vi "Datasheet Yield Result.vi"(6 "Connection Refnum":T1, 8 "error in (no error)":errorcluster, 10 "Yield Results":T3[](array[typedef]), 11 "Selected Test Type":string) -> (0 "error out":errorcluster, 3 "Key Array Out":T2)   [LabVIEW 2011]
uses:
  CGI Yield Results.ctl
  Addons/internet/utils/keyedarr.llb/Keyed Array.ctl
  SI.LIB/ODBC/SQL Controls/Connection Refnum.ctl
  Addons/internet/utils/strutil.llb/Case Matching.ctl
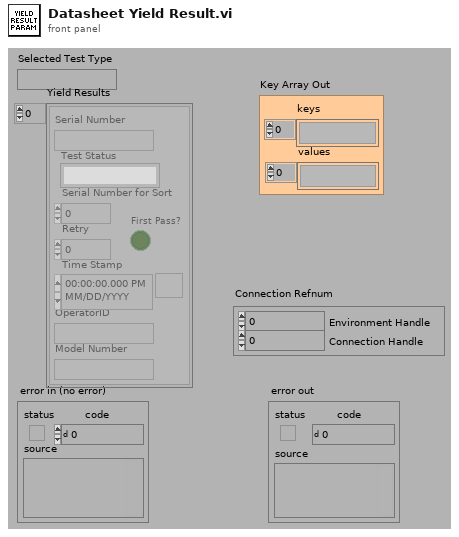
[diagram p1: front panel]
types:
  T1 = typedef "Connection Refnum.ctl" = cluster{"Environment Handle":i32, "Connection Handle":i32}
  T2 = typedef "Keyed Array.ctl" = cluster{"keys":string[], "values":string[]}
  T3 = typedef "CGI Yield Results.ctl" = cluster{"Model Number":string, "Serial Number for Sort":i32, "Serial Number":string, "Test Status":string, "Time Stamp":timestamp, "OperatorID":string, "Retry":i32, "First Pass?":bool}
  T4 = typedef "Case Matching.ctl" = enum16{"a != A", "a == A", "system"}
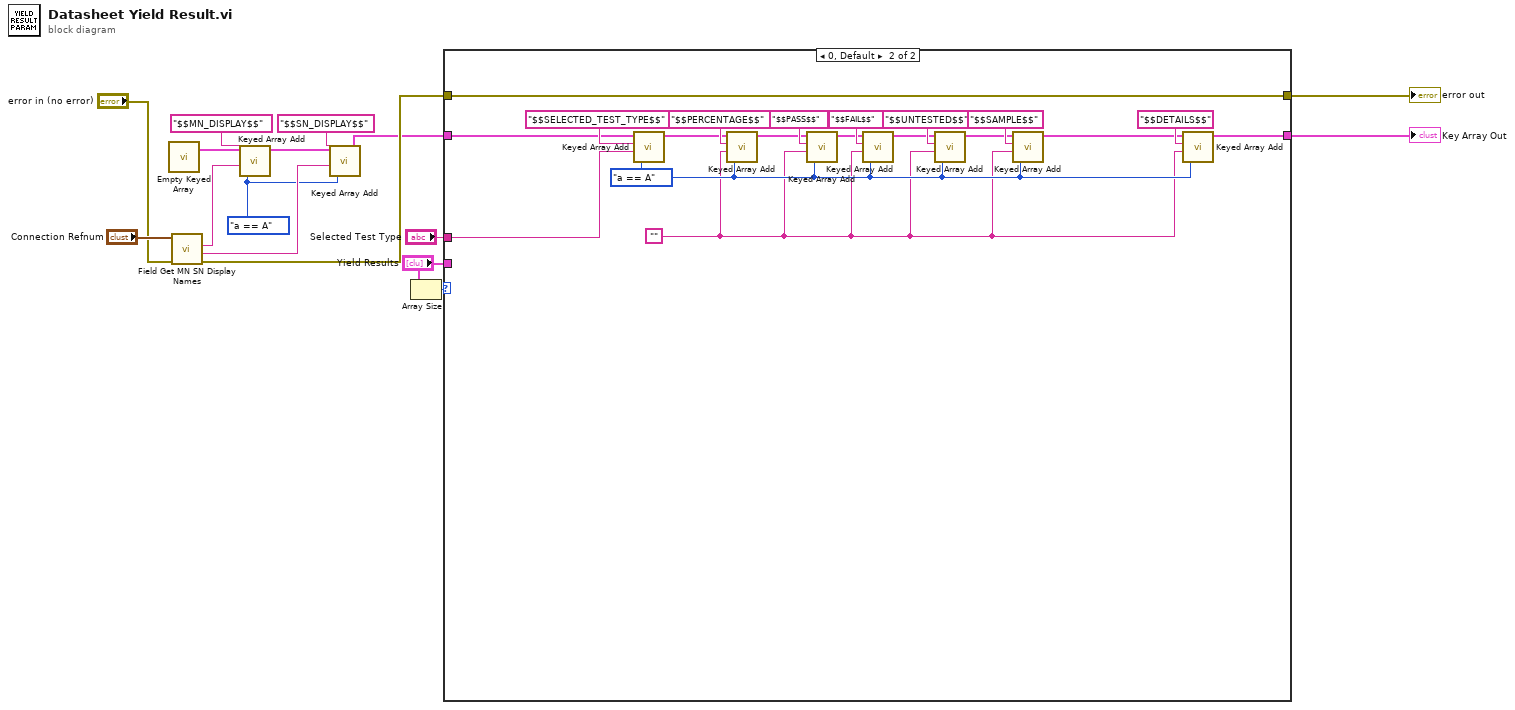
[diagram p0: block diagram]
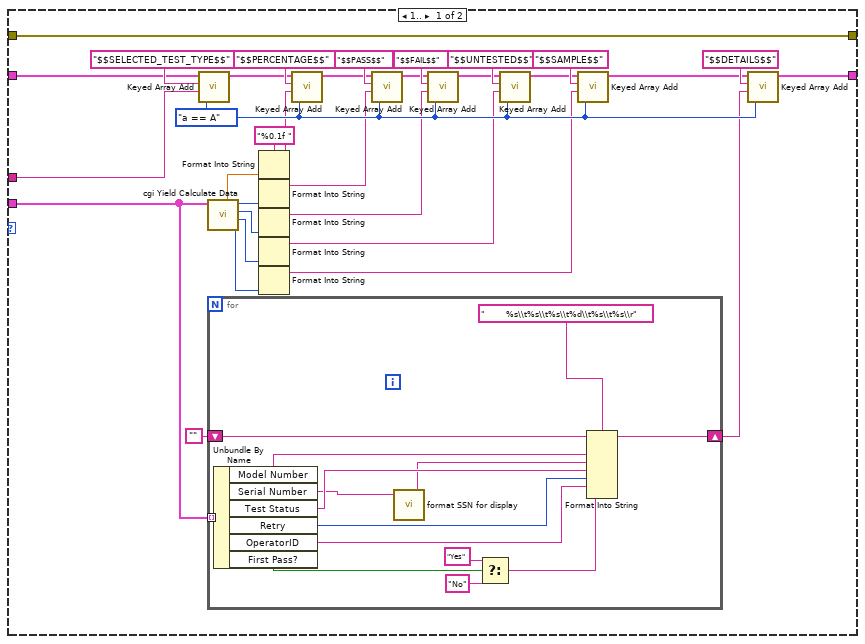
[diagram p2: hidden frame]
diagram:
  w6 = Case_Matching."a == A" ("case matching (sensitive)")
  n1 = call "Empty Keyed Array.vi"() -> ("empty keyed array"=w5:T2)  [unwired: 3 out]
  n2 = call "Field Get MN SN Display Names.vi"("error in (no error)"="error in (no error)", "Connection Refnum"="Connection Refnum") -> ("error out"=w2:errorcluster, "Serial Number Display Name"=w7:string, "Model Number Display Name"=w8:string)  [unwired: 7 out]
  n3 = call "Keyed Array Add.vi"("case matching (sensitive)"=w6, "value"=w8, "key"="$$MN_DISPLAY$$", "array in"=w5) -> ("array out"=w9:T2)  [unwired: 3 out]
  n4 = call "Keyed Array Add.vi"("case matching (sensitive)"=w6, "value"=w7, "key"="$$SN_DISPLAY$$", "array in"=w9) -> ("array out"=w1:T2)  [unwired: 3 out]
  n5 = Array Size(array="Yield Results") -> (size(s)=w14:i32)
  n6 = case shown="0, Default" w14 {
    tunnel: [w17 w64] -> w13
    tunnel: w2 -> [w17 w64]
    tunnel: [w18 w65] -> w12
    tunnel: "Selected Test Type" -> [w45 w78]
    tunnel: "Yield Results" -> [w22 _]
    tunnel: w1 -> [w19 w66]
    frame 1.. {
      w39 = Case_Matching."a == A" ("case matching (sensitive)")
      n7 = call "Keyed Array Add.vi"("case matching (sensitive)"=w39, "value"=w45, "key"="$$SELECTED_TEST_TYPE$$", "array in"=w19) -> ("array out"=w38:T2)  [unwired: 3 out]
      n8 = call "cgi Yield Calculate Data.vi"("Yield Results"=w22) -> ("# Sampled"=w24:i32, "# Untested"=w25:i32, "# Other"=w26:i32, "# Pass"=w27:i32, "Yield %"=w23:dbl)  [unwired: 6 out]
      n9 = for {
        tunnel: w22 -> [w62] mode=indexing
        shift-right: [w59] -> w20
        shift-left: "" -> [w58]
        n10 = Unbundle By Name(w62) -> ("Model Number"=w60:string, "Serial Number"=w55:string, "Test Status"=w57:string, "Retry"=w50:i32, "OperatorID"=w49:string, "First Pass?"=w52:bool)
        n11 = call "format SSN for display.vi"("string"=w55) -> ("s? t:f"=w54:string)  [unwired: 4 out]
        n12 = Select(t="Yes", s=w52, f="No") -> (s? t:f=w56:string)
        n13 = Format Into String(format string="       %s\\t%s\\t%s\\t%d\\t%s\\t%s\\r" ("string"), initial string=w58, w60, w54, w57, w50, w49, w56) -> (resulting string=w59:string)  [unwired: 1 in, 1 out]
      }
      n14 = Format Into String(format string="%0.1f ", w23) -> (resulting string=w32:string)  [unwired: 2 in, 1 out]
      n15 = Format Into String(w27) -> (resulting string=w31:string)  [unwired: 3 in, 1 out]
      n16 = Format Into String(w26) -> (resulting string=w30:string)  [unwired: 3 in, 1 out]
      n17 = Format Into String(w25) -> (resulting string=w29:string)  [unwired: 3 in, 1 out]
      n18 = Format Into String(w24) -> (resulting string=w28:string)  [unwired: 3 in, 1 out]
      n19 = call "Keyed Array Add.vi"("case matching (sensitive)"=w39, "value"=w32, "key"="$$PERCENTAGE$$", "array in"=w38) -> ("array out"=w37:T2)  [unwired: 3 out]
      n20 = call "Keyed Array Add.vi"("case matching (sensitive)"=w39, "value"=w31, "key"="$$PASS$$", "array in"=w37) -> ("array out"=w36:T2)  [unwired: 3 out]
      n21 = call "Keyed Array Add.vi"("case matching (sensitive)"=w39, "value"=w30, "key"="$$FAIL$$", "array in"=w36) -> ("array out"=w35:T2)  [unwired: 3 out]
      n22 = call "Keyed Array Add.vi"("case matching (sensitive)"=w39, "value"=w29, "key"="$$UNTESTED$$", "array in"=w35) -> ("array out"=w34:T2)  [unwired: 3 out]
      n23 = call "Keyed Array Add.vi"("case matching (sensitive)"=w39, "value"=w28, "key"="$$SAMPLE$$", "array in"=w34) -> ("array out"=w33:T2)  [unwired: 3 out]
      n24 = call "Keyed Array Add.vi"("case matching (sensitive)"=w39, "value"=w20, "key"="$$DETAILS$$", "array in"=w33) -> ("array out"=w18:T2)  [unwired: 3 out]
    }
    frame 0, Default {
      w63 = ""
      w73 = Case_Matching."a == A" ("case matching (sensitive)")
      n25 = call "Keyed Array Add.vi"("case matching (sensitive)"=w73, "value"=w78, "key"="$$SELECTED_TEST_TYPE$$", "array in"=w66) -> ("array out"=w72:T2)  [unwired: 3 out]
      n26 = call "Keyed Array Add.vi"("case matching (sensitive)"=w73, "value"=w63, "key"="$$PERCENTAGE$$", "array in"=w72) -> ("array out"=w71:T2)  [unwired: 3 out]
      n27 = call "Keyed Array Add.vi"("case matching (sensitive)"=w73, "value"=w63, "key"="$$PASS$$", "array in"=w71) -> ("array out"=w70:T2)  [unwired: 3 out]
      n28 = call "Keyed Array Add.vi"("case matching (sensitive)"=w73, "value"=w63, "key"="$$FAIL$$", "array in"=w70) -> ("array out"=w69:T2)  [unwired: 3 out]
      n29 = call "Keyed Array Add.vi"("case matching (sensitive)"=w73, "value"=w63, "key"="$$UNTESTED$$", "array in"=w69) -> ("array out"=w68:T2)  [unwired: 3 out]
      n30 = call "Keyed Array Add.vi"("case matching (sensitive)"=w73, "value"=w63, "key"="$$SAMPLE$$", "array in"=w68) -> ("array out"=w67:T2)  [unwired: 3 out]
      n31 = call "Keyed Array Add.vi"("case matching (sensitive)"=w73, "value"=w63, "key"="$$DETAILS$$", "array in"=w67) -> ("array out"=w65:T2)  [unwired: 3 out]
    }
  }
  "error out" <- w13
  "Key Array Out" <- w12
